vi "Cleanup.vi"(8 "error in (no error)":errorcluster, 11 "Abstract Message Rescripter in":refnum<class "Abstract Message Rescripter.lvclass">) -> (0 "error out":errorcluster, 3 "Abstract Message Rescripter out":refnum<class "Abstract Message Rescripter.lvclass">)   [LabVIEW 2020, in "Message Rescripter.lvlib" / "Abstract Message Rescripter.lvclass"]
uses:
  Abstract Message Rescripter.lvclass
  MessageMakerProvider/_Message Maker/_Maker Classes/Abstract Message Scripter/Abstract Message Scripter.lvclass
  Message Rescripter.lvlib
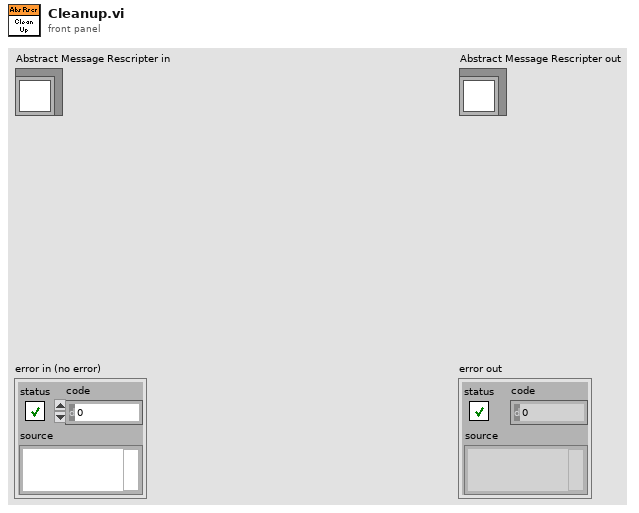
[diagram p1: front panel]
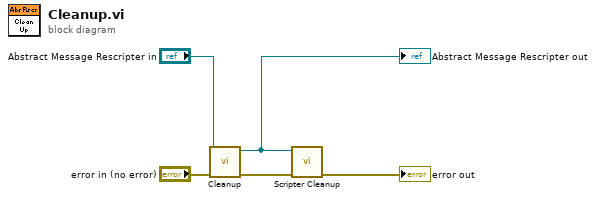
[diagram p0: block diagram]
diagram:
  n1 = call-parent "Cleanup.vi"("error in (no error)"="error in (no error)", "Message Scripter in"="Abstract Message Rescripter in") -> ("error out"=w3:errorcluster, "Message Scripter out"=w2:refnum<class "Abstract Message Rescripter.lvclass">)  [unwired: 8 in]
  "Abstract Message Rescripter out" <- w2
  n2 = call "Scripter Cleanup.vi"("error in (no error)"=w3, "Coupled Message Rescripter in"=w2) -> ("error out"=→"error out":errorcluster)  [unwired: 9 in]
